vi "Set TWM Corrections.vi"(4 "status ref (none)":refnum<vi>, 7 "Measurement properties":T1={"Measurement ID"=enum."1 signal, 1 ADC, 1 PJVS", "Description"="3 phase, 3 ADC, 1 PJVS", "Switching matrix M"=[], "Signal frequency  (Hz)"=50.0, "Maximal signal amplitude (V)"=0.0, "PRs (samples)"=0, "PRe (samples)"=0, "MRs (s)"=0.0, "MRe (s)"=0.0, "Set PJVS frequency (Hz)"=50.0, "PJVS reference voltages (1 period, V)"=[], "Requiested PJVS steps"=10, "Sampling f (Hz)"=7000.0, "Trigger mode"=enum."Trigger every MX switch", "Timing matrix (periods)"=[], "Record length (multiples of M)"=1, "Calculated"={"Triggers to next path (line of sequence)"=[], "Record samples"=0, "Sample indexes of switches"=[], "PRs (s)"=0.0, "PRe (s)"=0.0, "MRs (samples)"=0, "MRe (samples)"=0, "Trigger frequency  (Hz)"=50.0, "Measurement druation (s)"=0.0, "Samples per step"=0.0, "QPMX Sequence"=[], "PJVS segments frequency (Hz)"=50.0}, "No of required digitizers"=0, "No of required transducers"=0, "Transducer correction files"=[], "Digitizer correction file"=path "", "Algorithm"="TWM-PWRFFT"} {"Calculated"."Trigger frequency  (Hz)" format="%#_6p"; "Record length (multiples of M)" min=1 step=1; "PJVS reference voltages (1 period, V)" format="%.9g"; "MRe (s)" format="%#_4p"; "MRs (s)" format="%#_4p"}, 8 "error in":errorcluster, 11 "handle":i32) -> (0 "error out":errorcluster, 3 "handle out":i32)   [LabVIEW 2020]
doc: "Sets data processing in TWM. Sets algorithm and parameters."
uses:
  Type definitions/Measuement properties.ctl
  Type definitions/Measurement ID.ctl
  Type definitions/Trigger mode.ctl
  external libraries/TWM client.lvlibp/server/TWM client/TWM Client Transducer Correction Item.ctl
  external libraries/TWM client.lvlibp
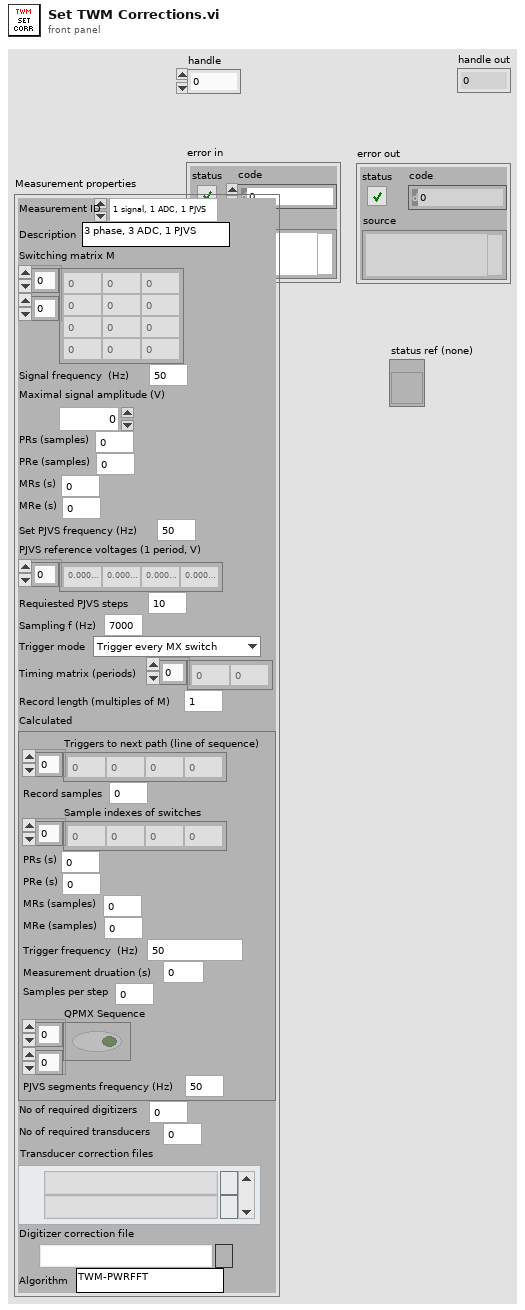
[diagram p1: front panel]
types:
  T1 = typedef "Measuement properties.ctl" = cluster{"Measurement ID":T2, "Description":string, "Switching matrix M":i32[][], "Signal frequency  (Hz)":dbl, "Maximal signal amplitude (V)":dbl, "PRs (samples)":u32, "PRe (samples)":u32, "MRs (s)":dbl, "MRe (s)":dbl, "Set PJVS frequency (Hz)":dbl, "PJVS reference voltages (1 period, V)":dbl[], "Requiested PJVS steps":u32, "Sampling f (Hz)":dbl, "Trigger mode":T3, "Timing matrix (periods)":i32[], "Record length (multiples of M)":u32, "Calculated":cluster{"Triggers to next path (line of sequence)":u32[], "Record samples":u32, "Sample indexes of switches":u32[], "PRs (s)":dbl, "PRe (s)":dbl, "MRs (samples)":i32, "MRe (samples)":i32, "Trigger frequency  (Hz)":dbl, "Measurement druation (s)":dbl, "Samples per step":dbl, "QPMX Sequence":bool[][], "PJVS segments frequency (Hz)":dbl}, "No of required digitizers":u32, "No of required transducers":u32, "Transducer correction files":path[], "Digitizer correction file":path, "Algorithm":string}
  T2 = typedef "Measurement ID.ctl" = enum16{"Manual setup", "1 signal, 1 ADC, 1 PJVS", "1 phase (U, I), 1 ADC, 1 PJVS", "1 phase (U, I), 2 ADC, 1 PJVS", "1 phase (U, I), 3 ADC, 1 PJVS", "3 phases (U1..3, I1..3), 3 ADC, 1 PJVS"}
  T3 = typedef "Trigger mode.ctl" = enum16{"Trigger every MX switch", "Trigger every sample"}
  T4 = typedef "TWM client.lvlibp/TWM Client Transducer Correction Item.ctl" = cluster{"path":path, "high ID":i32, "low ID":i32, "phase id":i32, "mux ID":i32}
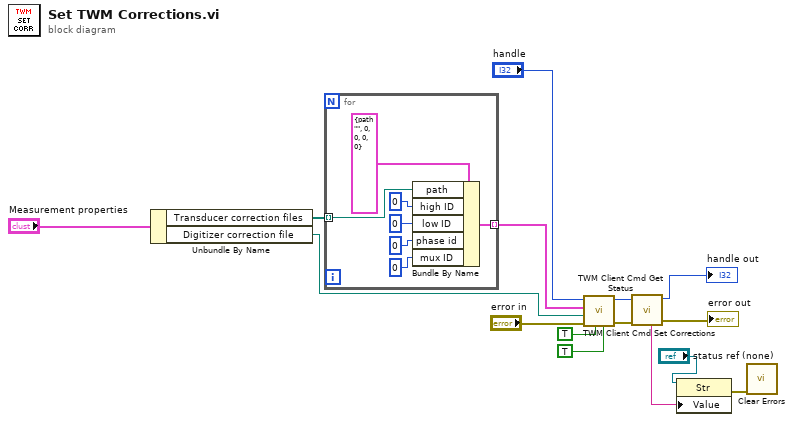
[diagram p0: block diagram]
diagram:
  n1 = Unbundle By Name("Measurement properties") -> ("Transducer correction files"=w9:path[], "Digitizer correction file"=w8:path)
  n2 = for {
    tunnel: [w21] -> w15 mode=indexing
    tunnel: w9 -> [w16] mode=indexing
    n3 = Bundle By Name(cluster=T4 {"path"=path "", "high ID"=0, "low ID"=0, "phase id"=0, "mux ID"=0} ("Cluster"), "path"=w16, "high ID"=0, "low ID"=0, "phase id"=0, "mux ID"=0) -> (w21:T4)
  }
  n4 = call "TWM Client Cmd Set Corrections.vi"("set digitizer (True)"=TRUE, "set transducers (True)"=TRUE, "error in"="error in", "digitizer correction"=w8, "list of transducers"=w15, "handle"="handle") -> ("error out"=w7:errorcluster, "handle out"=w5:i32)  [unwired: 4 in]
  n5 = call "TWM Client Cmd Get Status.vi"("error in"=w7, "handle"=w5) -> ("error out"=→"error out":errorcluster, "handle out"=→"handle out":i32, "status string"=w3:string)  [unwired: 5 in, 2 out]
  n6 = property class="Str"(reference="status ref (none)", "Value"=w3) -> (error out=w2:errorcluster)  [unwired: 1 in, 1 out]
  n7 = call <vilib>:"Clear Errors.vi"("error in (no error)"=w2) -> ()  [unwired: 5 in, 2 out]
